vi "CheckError.vi"(11 "Data string":string) -> (3 "T Error":bool)   [LabVIEW 2017]
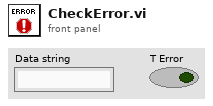
[diagram p1: front panel]
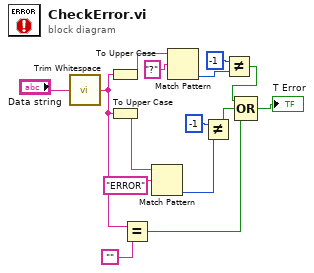
[diagram p0: block diagram]
diagram:
  n1 = call <vilib>:"Trim Whitespace.vi"("string"="Data string") -> ("trimmed string"=w2:string)  [unwired: 1 in]
  n2 = To Upper Case(1:w2) -> (0:w8:string)
  n3 = To Upper Case(1:w2) -> (0:w13:string)
  n4 = Equal?(x=w2, y="") -> (x = y?=w1:bool)
  n5 = Match Pattern(string=w13, regular expression="ERROR" ("y")) -> (offset past match=w10:i32)  [unwired: 1 in, 3 out]
  n6 = Match Pattern(string=w8, regular expression="?" ("y")) -> (offset past match=w5:i32)  [unwired: 1 in, 3 out]
  n7 = Not Equal?(x=-1, y=w10) -> (x != y?=w11:bool)
  n8 = Not Equal?(x=-1, y=w5) -> (x != y?=w4:bool)
  n9 = Compound Arithmetic op=OR(w4, w11, w1) -> (→"T Error":bool)
